vi "Configure Laser AO.vi"(8 "error in":errorcluster, 11 "cCRDS in":refnum<class "cCRDS.lvclass">=refnum) -> (0 "error out":errorcluster, 3 "cCRDS out":refnum<class "cCRDS.lvclass">)   [LabVIEW 2015, in "cCRDS.lvclass"]
uses:
  cCRDS.lvclass
  cCRDS.lvclass/cCRDS.ctl
  <vilib>/DAQmx/write.llb/DAQmx Write (Digital 1D Bool NChan 1Samp 1Line).vi
  <vilib>/DAQmx/miscellaneous.llb/DAQmx Fill In Error Info.vi
  <vilib>/DAQmx/configure/timing.llb/DAQmx Timing (Implicit).vi
  <vilib>/DAQmx/configure/trigger.llb/DAQmx Start Trigger (Digital Edge).vi
  Data Access/Write Laser Out.vi
  <resource>/objmgr/daqmx.rc
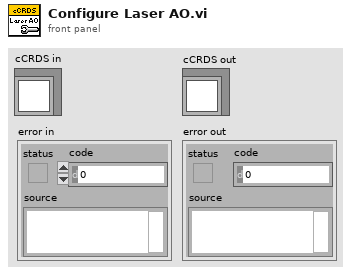
[diagram p1: front panel]
types:
  T1 = cluster{"YAG CO":refnum<k21>, "LaserEn":refnum<k21>, "Diode CO":refnum<k21>}
  T2 = cluster{"[0]":bool, "[1]":bool, "[2]":bool, "[3]":bool}
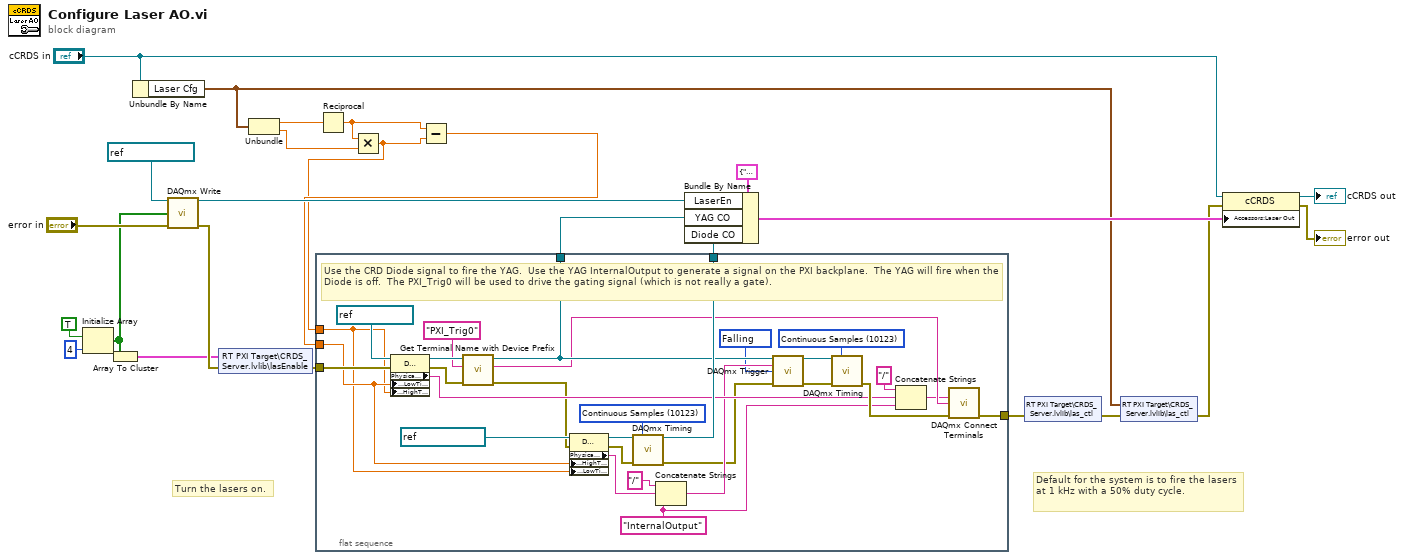
[diagram p0: block diagram]
diagram:
  # "Turn the lasers on."
  # "Default for the system is to fire the lasers at 1 kHz with a 50% duty cycle."
  n1 = Initialize Array(TRUE, 4 ("dimension size")) -> (w18:bool[])
  n2 = Array To Cluster(array=w18) -> (cluster=w19:T2)
  n3 = Unbundle By Name("cCRDS in") -> ("Laser Cfg"=w6:cluster{"Rate (Hz)":sgl, "DC (%)":sgl})
  n4 = call-poly <vilib>:"DAQmx Write.vi"("task/channels in"=refnum<k21> "CRD Las En" ("Laser AI"), "data"=w18, "error in"="error in") -> ("task out"=w14:refnum<k21>, "error out"=w20:errorcluster)  [unwired: 10 in, 1 out]
  n5 = shared-variable "RT PXI Target\\CRDS_Server.lvlib\\lasEnable"(w19, error in=w20) -> (error out=w11:errorcluster)
  n6 = Unbundle(w6) -> ("Rate (Hz)"=w5:sgl, "DC (%)"=w4:sgl)
  n7 = flat-sequence {
    tunnel: [w53] -> w24
    tunnel: [w52] -> w23
    tunnel: w11 -> [w33]
    tunnel: [w30] -> w9
    tunnel: w2 -> [w27]
    tunnel: w1 -> [w26]
    frame #0 {
      w46 = "InternalOutput" ("string")
      w36 = 10123 items=["Finite Samples"=10178, "Continuous Samples"=10123, "Hardware Timed Single Point"=12522] ("sample mode")
      w35 = 10123 items=["Finite Samples"=10178, "Continuous Samples"=10123, "Hardware Timed Single Point"=12522] ("sample mode")
      w34 = 10171 items=["Rising"=10280, "Falling"=10171] ("edge")
      # "Use the CRD Diode signal to fire the YAG.  Use the YAG InternalOutput to generate a signal on the PXI backplane.  The YAG will fire when the Diode is off.  The PXI_Trig0 will be used to drive the gating signal (which is not really a gate)."
      n8 = property class="DAQmx Channel"(reference=refnum<k21> "CRD YAG" ("YAG CO"), error in=w33, "CO.Pulse.LowTime"=w27, "CO.Pulse.HighTime"=w26) -> (reference out=w45:refnum<k21>, error out=w49:errorcluster, "PhysicalChanName"=w44:tag)
      n9 = call "Get Terminal Name with Device Prefix.vi"("error in"=w49, "Local Terminal Name"="PXI_Trig0", "task/channels in"=w45) -> ("error out"=w32:errorcluster, "Terminal Name with Device Prefix"=w48:tag, "task out"=w52:refnum<k21>)  [unwired: 6 in]
      n10 = property class="DAQmx Channel"(reference=refnum<k21> "CRD Diode" ("Diode CO"), error in=w32, "CO.Pulse.HighTime"=w27, "CO.Pulse.LowTime"=w26) -> (reference out=w38:refnum<k21>, error out=w50:errorcluster, "PhysicalChanName"=w39:tag)
      n11 = call-poly <vilib>:"DAQmx Timing.vi"("task/channels in"=w38, "sample mode"=w36, "error in"=w50) -> ("task out"=w53:refnum<k21>, "error out"=w31:errorcluster)  [unwired: 11 in]
      n12 = Concatenate Strings("/", w39, w46) -> (w40:string)
      n13 = call-poly <vilib>:"DAQmx Trigger.vi"("task/channels in"=w52, "source"=w40, "edge"=w34, "error in"=w31) -> ("task out"=w29:refnum<k21>, "error out"=w51:errorcluster)  [unwired: 10 in]
      n14 = call-poly <vilib>:"DAQmx Timing.vi"("task/channels in"=w29, "sample mode"=w35, "error in"=w51) -> ("error out"=w54:errorcluster)  [unwired: 11 in, 1 out]
      n15 = Concatenate Strings("/", w44, w46) -> (w43:string)
      n16 = call <vilib>:"DAQmx Connect Terminals.vi"("source terminal"=w43, "destination terminal"=w48, "error in"=w54) -> ("error out"=w30:errorcluster)  [unwired: 12 in]
    }
  }
  n17 = Reciprocal(x=w5) -> (1/x=w3:sgl)
  n18 = Multiply(x=w3, y=w4) -> (x*y=w1:sgl)
  n19 = Subtract(x=w3, y=w1) -> (x-y=w2:sgl)
  n20 = Bundle By Name(cluster=T1 {"YAG CO"="CRD YAG", "LaserEn"="CRD Las En", "Diode CO"="CRD Diode"} ("Laser Out"), "LaserEn"=w14, "YAG CO"=w23, "Diode CO"=w24) -> (w15:T1)
  n21 = shared-variable "RT PXI Target\\CRDS_Server.lvlib\\las_ctl"(error in=w9) -> (error out=w10:errorcluster)  [unwired: 1 out]
  n22 = shared-variable "RT PXI Target\\CRDS_Server.lvlib\\las_ctl"(w6, error in=w10) -> (error out=w8:errorcluster)
  n23 = property class="cCRDS"(reference="cCRDS in", error in=w8, "Accessors:Laser Out"=w15) -> (reference out=→"cCRDS out":refnum<class "cCRDS.lvclass">, error out=→"error out":errorcluster)
